vi "celsius to Fahrenheit with warning message dialog box.vi"() -> ()   [LabVIEW 2019]
panel:
  out "warning":bool
  out "celsius":dbl
  out "Fahrenheit":dbl(slide) scale=0.0..300.0
  in  "celsius":dbl(knob) scale=0.0..150.0
  out "Fahrenheit":dbl
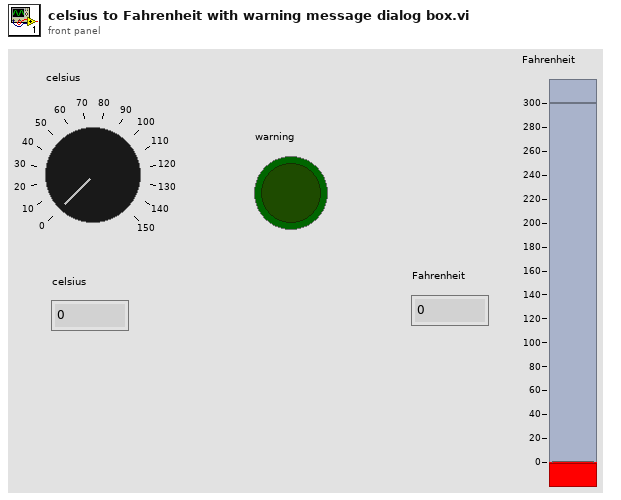
[diagram p1: front panel]
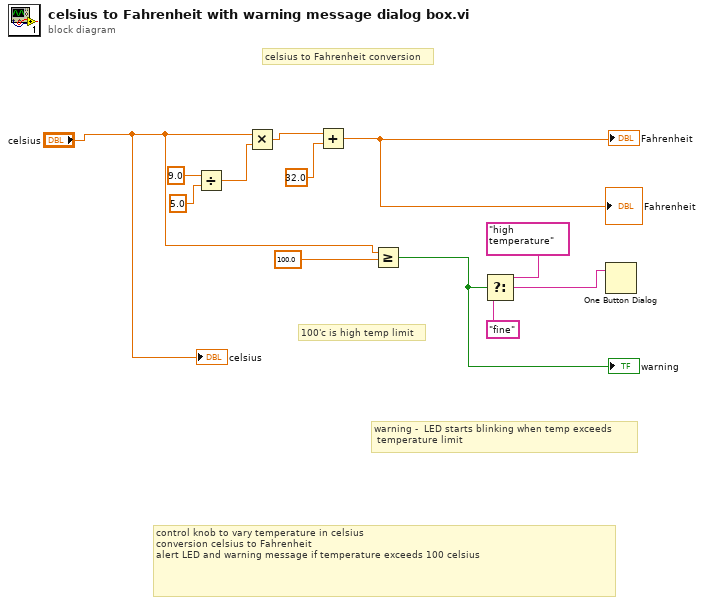
[diagram p0: block diagram]
diagram:
  # "control knob to vary temperature in celsius \nconversion celsius to Fahrenheit\nalert LED and warning message if temperature exceeds 100 celsius"
  # "celsius to Fahrenheit conversion"
  # "warning -  LED starts blinking when temp exceeds\n temperature limit"
  # "100'c is high temp limit"
  n1 = Divide(x=9.0, y=5.0) -> (x/y=w10:dbl)
  n2 = Multiply(x="celsius", y=w10) -> (x*y=w9:dbl)
  n3 = Add(x=w9, y=32.0) -> (x+y=→"Fahrenheit" →"Fahrenheit":dbl)
  n4 = Greater Or Equal?(x="celsius", y=100.0) -> (x >= y?=w1:bool)
  "warning" <- w1
  n5 = Select(t="high temperature", s=w1, f="fine") -> (s? t:f=w6:string)
  n6 = One Button Dialog(message=w6) -> ()  [unwired: 1 in, 1 out]
  "celsius" <- "celsius"
